vi "joystik FGV.vi"() -> ()   [LabVIEW 2019]
uses:
  <vilib>/Utility/inputDevices.llb/joystickAcquire.vi
  <vilib>/Utility/inputDevices.llb/closeJoystick.vi
panel:
  out "error out":errorcluster
  in  "stop":bool
  out "axis info":T1
  out "button info":T2
  out "direction info":T3
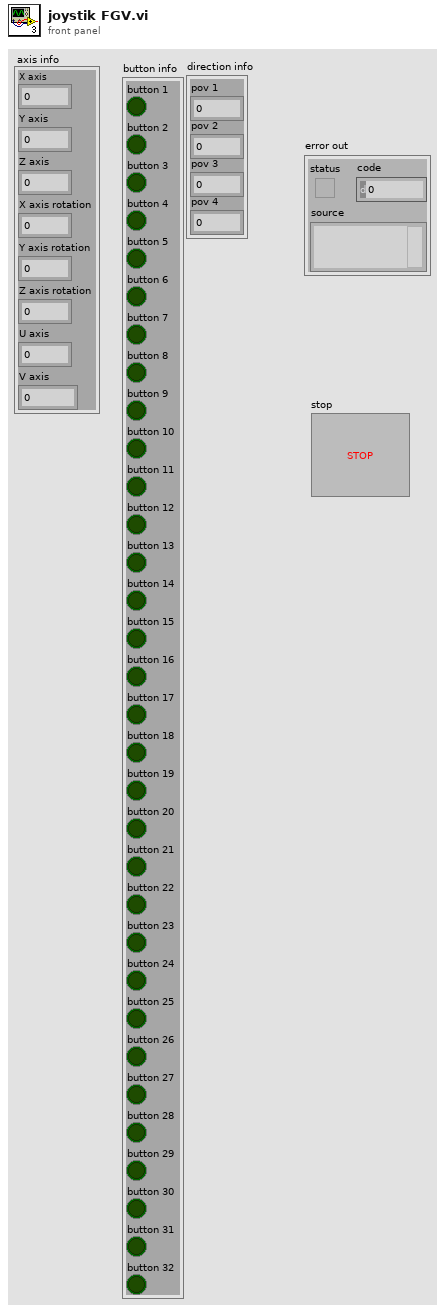
[diagram p1: front panel]
types:
  T1 = cluster{"X axis":i32, "Y axis":i32, "Z axis":i32, "X axis rotation":i32, "Y axis rotation":i32, "Z axis rotation":i32, "U axis":i32, "V axis":i32}
  T2 = cluster{"button 1":bool, "button 2":bool, "button 3":bool, "button 4":bool, "button 5":bool, "button 6":bool, "button 7":bool, "button 8":bool, "button 9":bool, "button 10":bool, "button 11":bool, "button 12":bool, "button 13":bool, "button 14":bool, "button 15":bool, "button 16":bool, "button 17":bool, "button 18":bool, "button 19":bool, "button 20":bool, "button 21":bool, "button 22":bool, "button 23":bool, "button 24":bool, "button 25":bool, "button 26":bool, "button 27":bool, "button 28":bool, "button 29":bool, "button 30":bool, "button 31":bool, "button 32":bool}
  T3 = cluster{"pov 1":i32, "pov 2":i32, "pov 3":i32, "pov 4":i32}
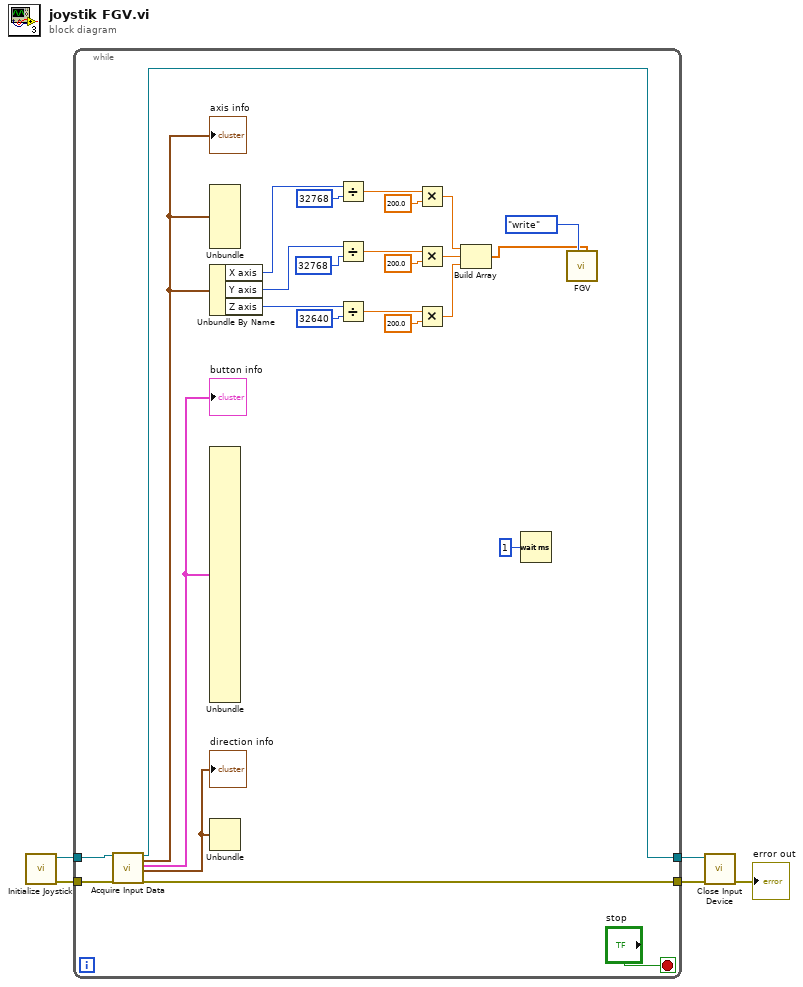
[diagram p0: block diagram]
diagram:
  n1 = call <vilib>:"Initialize Joystick.vi"() -> ("error out"=w2:errorcluster, "device ID"=w5:refnum<k1>)  [unwired: 10 in]
  n2 = while {
    tunnel: [w30] -> w3
    tunnel: [w29] -> w4
    tunnel: w5 -> [w10]
    tunnel: w2 -> [w9]
    stop <- "stop" stop-if-true
    n3 = call-poly <vilib>:"Acquire Input Data.vi"("device ID"=w10, "error in (no error)"=w9) -> ("device ID"=w29:refnum<k1>, "axis info"=w26:T1, "button info"=w28:T2, "direction info"=w27:T3, "error out"=w30:errorcluster)  [unwired: 13 in]
    "axis info" <- w26
    "button info" <- w28
    "direction info" <- w27
    n4 = Unbundle(w26) -> ()  [unwired: 8 out]
    n5 = Unbundle By Name(w26) -> ("X axis"=w25:i32, "Y axis"=w24:i32, "Z axis"=w23:i32)
    n6 = Unbundle(w28) -> ()  [unwired: 32 out]
    n7 = Unbundle(w27) -> ()  [unwired: 4 out]
    n8 = Divide(x=w25, y=32768) -> (x/y=w19:dbl)
    n9 = Divide(x=w24, y=32768) -> (x/y=w17:dbl)
    n10 = Divide(x=w23, y=32640) -> (x/y=w15:dbl)
    n11 = Multiply(x=w19, y=200.0) -> (x*y=w13:dbl)
    n12 = Multiply(x=w17, y=200.0) -> (x*y=w12:dbl)
    n13 = Multiply(x=w15, y=200.0) -> (x*y=w11:dbl)
    n14 = Build Array(w13, w12, w11) -> (w6:dbl[])
    n15 = Wait (ms)(milliseconds to wait=u32 1) -> ()  [unwired: 1 out]
    n16 = call "FGV.vi"("write"=w6, "action"=enum16{"read", "write"}."write") -> ()  [unwired: 9 in, 1 out]
  }
  n17 = call-poly <vilib>:"Close Input Device.vi"("error in (no error)"=w3, "device ID"=w4) -> ("error out"=→"error out":errorcluster)  [unwired: 8 in]
